vi "GetBars.vi"(8 "error in (no error)":errorcluster, 10 "Munged Input":string, 11 "EAN-13 in":refnum<class "EAN-13.lvclass">) -> (0 "error out":errorcluster, 2 "BarWidths":T1[][](array[typedef]), 3 "EAN-13 out":refnum<class "EAN-13.lvclass">)   [LabVIEW 2013, in "BarCodes.lvlib" / "EAN-13.lvclass"]
doc: "Gets the bars of the bar code. The bars are specified as an array of bar widths from left to right."
uses:
  EAN-13.lvclass
  BarCode/Bar.ctl
  BarCode/BarCode.lvclass
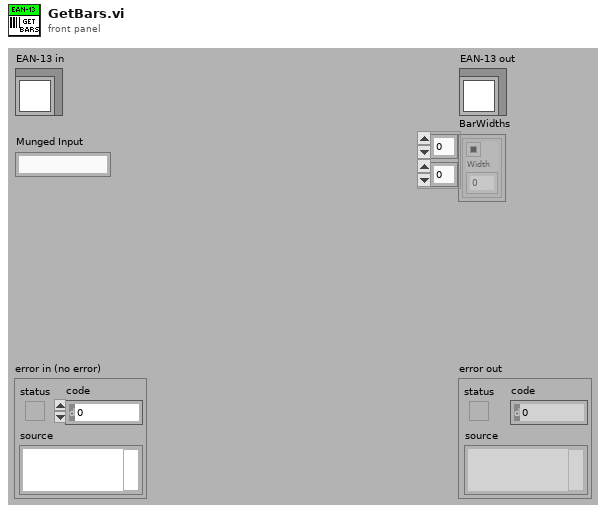
[diagram p1: front panel]
types:
  T1 = typedef "BarCodes.lvlib/BarCode.lvclass/Bar.ctl" = cluster{"Color":u32, "Width":u8}
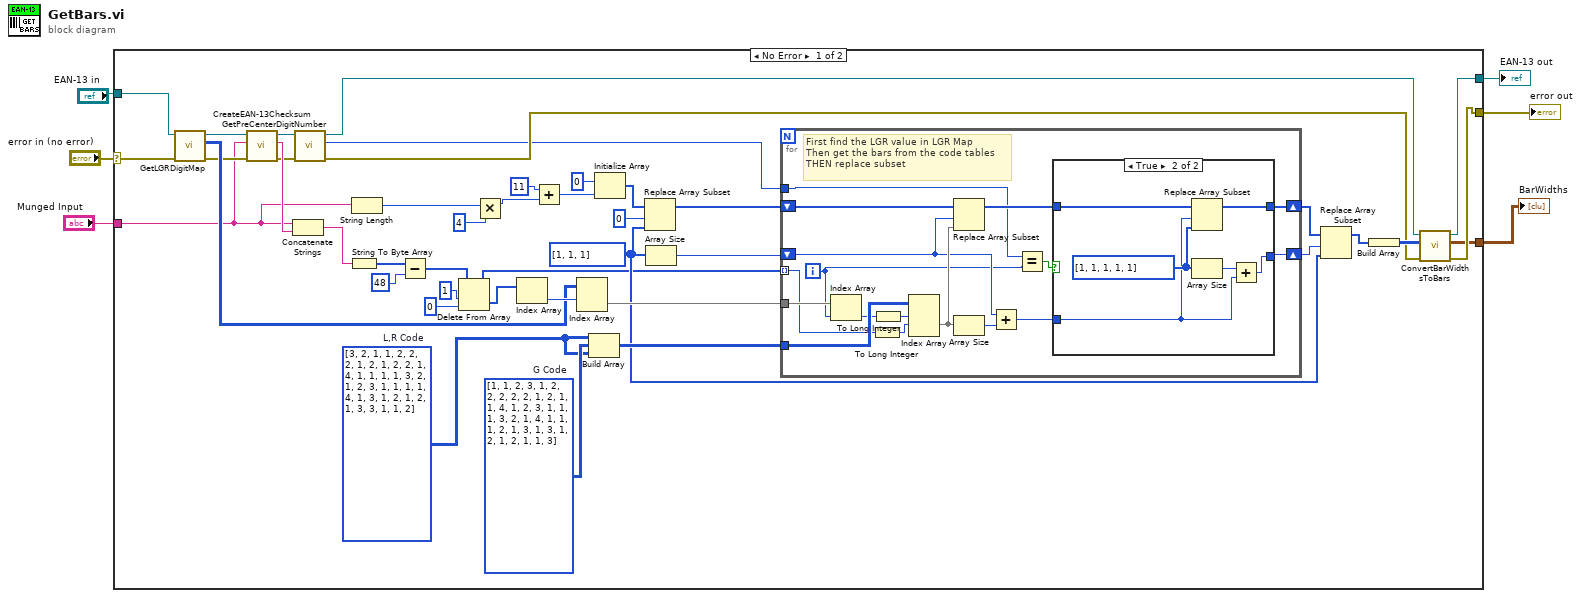
[diagram p0: block diagram]
diagram:
  n1 = case shown="No Error" "error in (no error)" {
    selector: "error in (no error)" -> [w15 w75]
    tunnel: "EAN-13 in" -> [w14 w76]
    tunnel: [w20 w76] -> w5
    tunnel: "Munged Input" -> [w7 _]
    tunnel: [w19 w75] -> w2
    tunnel: [w18 _] -> w1
    frame No Error {
      w33 = u8[] [1, 1, 1]
      w47 = u8[][] [[1, 1, 2, 3], [1, 2, 2, 2], [2, 2, 1, 2], [1, 1, 4, 1], [2, 3, 1, 1], [1, 3, 2, 1], [4, 1, 1, 1], [2, 1, 3, 1], [3, 1, 2, 1], [2, 1, 1, 3]]  # G Code
      w23 = u8[][] [[3, 2, 1, 1], [2, 2, 2, 1], [2, 1, 2, 2], [1, 4, 1, 1], [1, 1, 3, 2], [1, 2, 3, 1], [1, 1, 1, 4], [1, 3, 1, 2], [1, 2, 1, 3], [3, 1, 1, 2]]  # L,R Code
      n2 = call-dynamic "GetLGRDigitMap.vi"("error in (no error)"=w15, "EAN-13 in"=w14) -> ("error out"=w16:errorcluster, "LGR digit map"=w17:u8[][], "EAN-13 out"=w13:refnum<class "EAN-13.lvclass">)  [unwired: 7 in]
      n3 = call "CreateEAN-13Checksum.vi"("error in (no error)"=w16, "String"=w7, "EAN-13 in"=w13) -> ("error out"=w12:errorcluster, "Checksum"=w31:string, "EAN-13 out"=w11:refnum<class "EAN-13.lvclass">)  [unwired: 6 in]
      n4 = Concatenate Strings(w7, w31) -> (w30:string)
      n5 = call-dynamic "GetPreCenterDigitNumber.vi"("error in (no error)"=w12, "EAN-13 in"=w11) -> ("error out"=w9:errorcluster, "Numeric"=w8:i32, "EAN-13 out"=w10:refnum<class "EAN-13.lvclass">)  [unwired: 7 in]
      n6 = String To Byte Array(string=w30) -> (unsigned byte array=w49:u8[])
      n7 = String Length(string=w7) -> (length=w29:i32)
      n8 = Subtract(x=w49, y=u8 48) -> (x-y=w26:u8[])
      n9 = Delete From Array(array=w26, length=1, index=0) -> (deleted portion=w27:u8[], array with subset deleted=w25:u8[])
      n10 = Multiply(x=w29, y=4) -> (x*y=w37:i32)
      n11 = Index Array(array=w27) -> (element=w48:u8)  [unwired: 1 in]
      n12 = Add(x=11, y=w37) -> (x+y=w43:i32)
      n13 = Index Array(array=w17, index (row)=w48) -> (element=w45:u8[])  [unwired: 1 in]
      n14 = Build Array(w23, w47, w23) -> (w46:u8[][][])
      n15 = Initialize Array(u8 0, w43) -> (w41:u8[])
      n16 = Replace Array Subset(array=w41, new element=w33, index=0) -> (w40:u8[])
      n17 = Array Size(array=w33) -> (size(s)=w38:i32)
      n18 = for {
        tunnel: w25 -> [w63] mode=indexing
        tunnel: w46 -> [w65]
        tunnel: w45 -> [w66]
        shift-right: [w56] -> w35
        shift-left: w40 -> [w62]
        shift-right: [w55] -> w34
        shift-left: w38 -> [w59]
        tunnel: w8 -> [w51]
        i -> [w52]
        # "First find the LGR value in LGR Map\nThen get the bars from the code tables\nTHEN replace subset"
        n19 = Index Array(array=w66, index=w52) -> (element=w64:u8)
        n20 = To Long Integer(number=w63) -> (32bit integer=w53:i32)
        n21 = To Long Integer(number=w64) -> (32bit integer=w54:i32)
        n22 = Index Array(array=w65, index (dim 0)=w54, index (dim 1)=w53) -> (element=w60:u8[])  [unwired: 1 in]
        n23 = Replace Array Subset(array=w62, new element=w60, index=w59) -> (w61:u8[])
        n24 = Array Size(array=w60) -> (size(s)=w58:i32)
        n25 = Add(x=w59, y=w58) -> (x+y=w57:i32)
        n26 = Equal?(x=w51, y=w52) -> (x = y?=w50:bool)
        n27 = case shown="True" w50 {
          tunnel: w61 -> [w68 w74]
          tunnel: w57 -> [w67 w70]
          tunnel: [w68 w73] -> w56
          tunnel: [w67 w69] -> w55
          frame False {
          }
          frame True {
            w72 = u8[] [1, 1, 1, 1, 1]
            n28 = Replace Array Subset(array=w74, new element=w72, index=w70) -> (w73:u8[])
            n29 = Array Size(array=w72) -> (size(s)=w71:i32)
            n30 = Add(x=w71, y=w70) -> (x+y=w69:i32)
          }
        }
      }
      n31 = Replace Array Subset(array=w35, new element=w33, index=w34) -> (w22:u8[])
      n32 = Build Array(w22) -> (w21:u8[][])
      n33 = call "ConvertBarWidthsToBars.vi"("error in (no error)"=w9, "BarWidths"=w21, "BarCode in"=w10) -> ("error out"=w19:errorcluster, "Bars"=w18:T1[][], "BarCode out"=w20:refnum<class "EAN-13.lvclass">)  [unwired: 6 in]
    }
    frame Error {
    }
  }
  "error out" <- w2
  "EAN-13 out" <- w5
  "BarWidths" <- w1
